vi "Convert serial string to Eng vals.vi"(0 "Serial buffer string (excluding FrameChar)":string) -> (3 "Pressures":sgl[][](graph), 6 "External thermistor temperature (deg C)":sgl, 8 "Sensor die temperatures (deg C)":sgl[](array[numeric]), 13 "All vals":sgl[](array[numeric]))   [LabVIEW 2017]
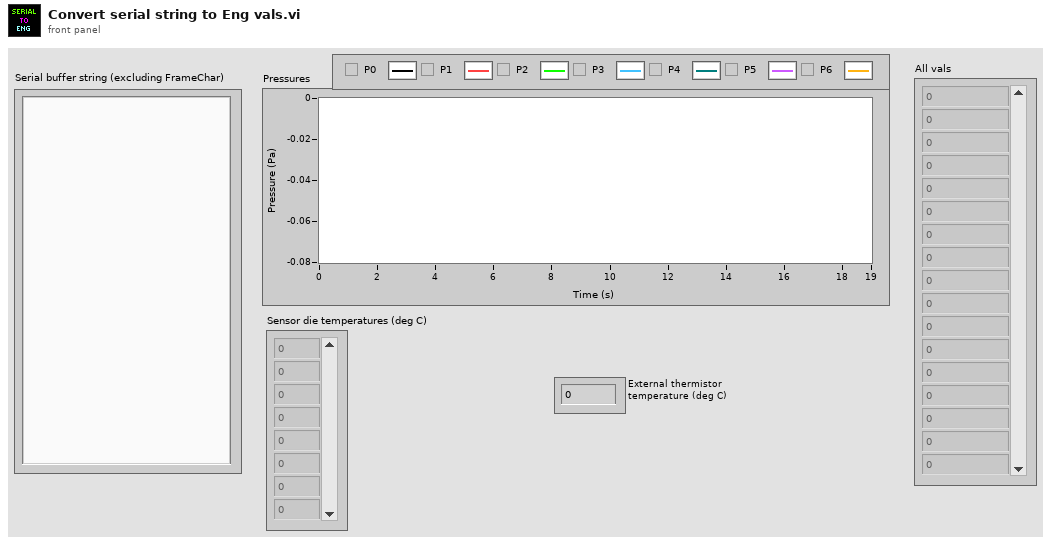
[diagram p1: front panel]
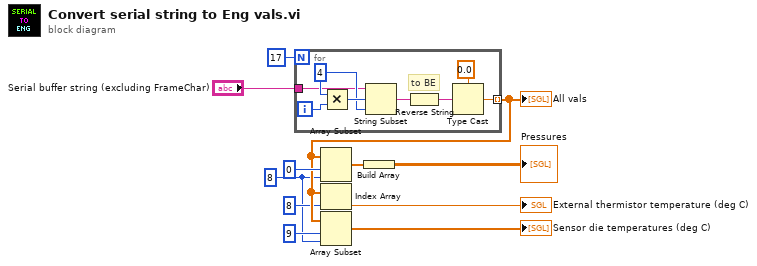
[diagram p0: block diagram]
diagram:
  w1 = 8 ("length")
  n1 = for {
    N: 17 -> [_]
    tunnel: [w13] -> w5 mode=indexing
    tunnel: "Serial buffer string (excluding FrameChar)" -> [w12]
    i -> [w19]
    w17 = 4 ("x")
    # "to BE"
    n2 = Multiply(x=w17, y=w19) -> (x*y=w18:i32)
    n3 = String Subset(string=w12, offset (0)=w18, length (rest)=w17) -> (substring=w16:string)
    n4 = Reverse String(1:w16) -> (0:w15:string)
    n5 = Type Cast(type=sgl 0.0 ("byte count"), x=w15) -> (*(type *) &x=w13:sgl)
  }
  "All vals" <- w5
  n6 = Array Subset(array=w5, index=0, length=w1) -> (w8:sgl[])
  n7 = Index Array(array=w5, index=8) -> (element=→"External thermistor temperature (deg C)":sgl)
  n8 = Array Subset(array=w5, index=9, length=w1) -> (→"Sensor die temperatures (deg C)":sgl[])
  n9 = Build Array(w8) -> (→"Pressures":sgl[][])
